vi "execution class name.vi"(8 "error in":errorcluster, 11 "configuration in":refnum<class "CVT Engine Configuration.lvclass">) -> (0 "error out":errorcluster, 2 "execution class":string, 3 "configuration out":refnum<class "CVT Engine Configuration.lvclass">)   [LabVIEW 2013, in "CVT Engine Configuration.lvclass"]
uses:
  CVT Engine Configuration.lvclass
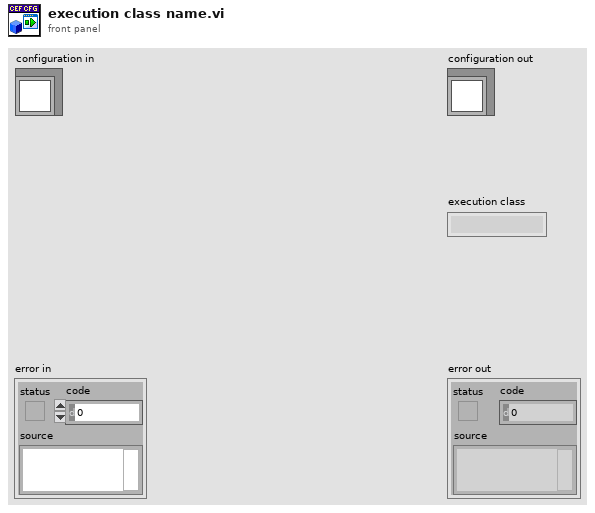
[diagram p1: front panel]
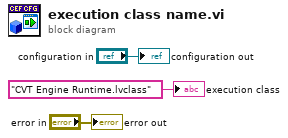
[diagram p0: block diagram]
diagram:
  "error out" <- "error in"
  "configuration out" <- "configuration in"
  "execution class" <- "CVT Engine Runtime.lvclass" ("execution class")
